vi "Set_stepcount.vi"(8 "error in (no error)":errorcluster, 10 "Set_stepcount":i32, 11 "connection ID":refnum<k5>) -> (0 "error out":errorcluster, 3 "TCP Network Connection out":refnum<k5>)   [LabVIEW 2019]
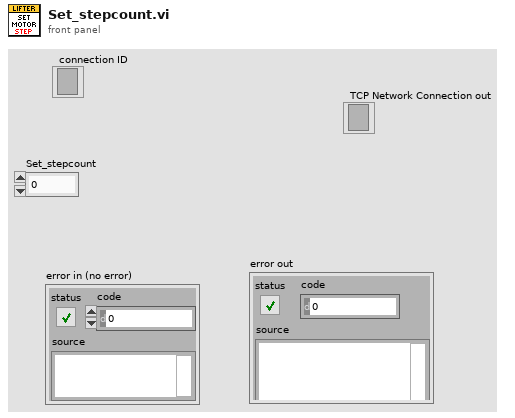
[diagram p1: front panel]
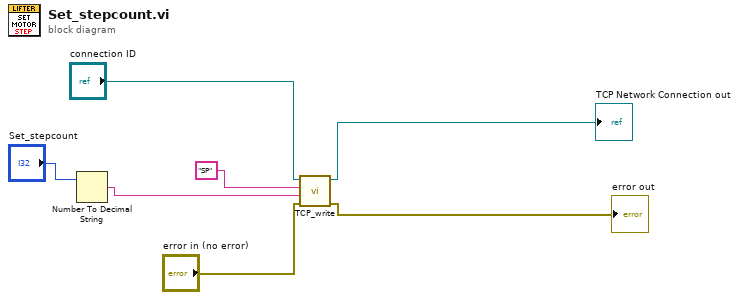
[diagram p0: block diagram]
diagram:
  n1 = Number To Decimal String(number="Set_stepcount") -> (decimal integer string=w5:string)  [unwired: 1 in]
  n2 = call "TCP_write.vi"("error in"="error in (no error)", "Parameter 2"=w5, "Parameter 1"="SP" ("string"), "connection ID"="connection ID") -> ("error out"=→"error out":errorcluster, "TCP Network Connection out"=→"TCP Network Connection out":refnum<k5>)  [unwired: 5 in, 1 out]
